vi "Set Inst Mode.vi"(8 "error in (no error)":errorcluster, 10 "ABS/INC":bool, 11 "FujiMotor in":refnum<class "FujiMotor.lvclass">) -> (0 "error out":errorcluster, 3 "FujiMotor out":refnum<class "FujiMotor.lvclass">)   [LabVIEW 2014, in "ALPHA5 RS485.lvlib" / "FujiMotor.lvclass"]
uses:
  FujiMotor.lvclass
  FujiMotor.lvclass/FujiMotor.ctl
  ALPHA5 RS485.lvlib
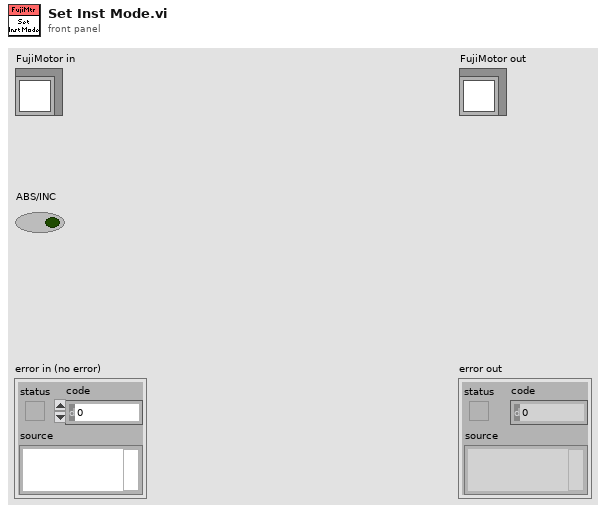
[diagram p1: front panel]
types:
  T1 = typedef "ALPHA5 RS485.lvlib/Port Selection Info.ctl" = cluster{"Port Name":refnum<visa-resource-name>, "Amplifier Num":u8, "Baud Rate":u32, "Char Formation":enum16{"0", "1", "2", "3", "4", "5"}}
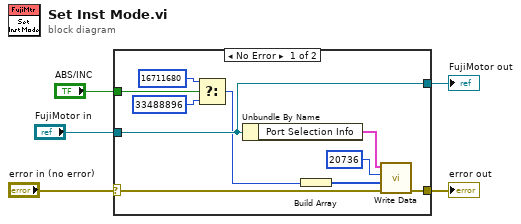
[diagram p0: block diagram]
diagram:
  n1 = case shown="No Error" "error in (no error)" {
    selector: "error in (no error)" -> [w7 w16]
    tunnel: [w6 w16] -> w4
    tunnel: [w15 w17] -> w2
    tunnel: "FujiMotor in" -> [w15 w17]
    tunnel: "ABS/INC" -> [w12 _]
    frame No Error {
      n2 = Select(t=16711680 ("Numeric"), s=w12, f=33488896 ("Numeric")) -> (s? t:f=w9:i32)
      n3 = Unbundle By Name(w15) -> ("Port Selection Info"=w14:T1)
      n4 = Build Array(w9) -> (w8:i32[])
      n5 = call "Write Data.vi"("error in (no error)"=w7, "Data"=w8, "Address"=u16 20736, "Port Selection Info In"=w14) -> ("error out"=w6:errorcluster)  [unwired: 6 in, 1 out]
    }
    frame Error {
    }
  }
  "error out" <- w4
  "FujiMotor out" <- w2
